vi "2500A and Neocera.vi"() -> ()   [LabVIEW 2010]
uses:
  <vilib>/Utility/file.llb/Write To Spreadsheet File (DBL).vi
  <vilib>/ptbypt/NI_PtbyPt.lvlib
panel:
  in  "AH2500A  GPIB":refnum<visa-resource-name>
  in  "Neocera GPIB":refnum<visa-resource-name>
  in  "Number of\n data points\nto average":i32
  out "Temperature":dbl format="%.3f"
  in  "Save?":bool
  in  "file path (dialog if empty)":path
  out "XY Graph":cluster{dbl[], dbl[]}(graph)
  out "Capacitance":ext format="%#.6g"
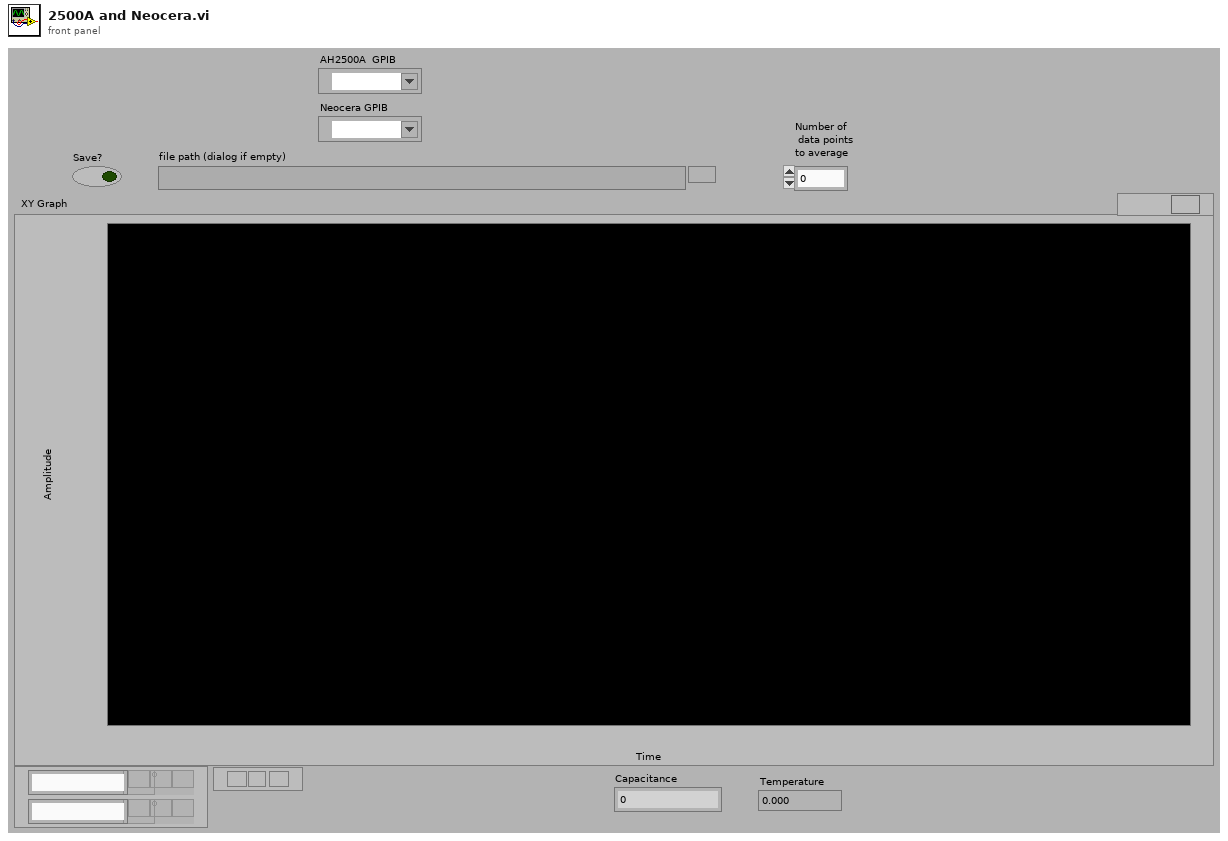
[diagram p1: front panel]
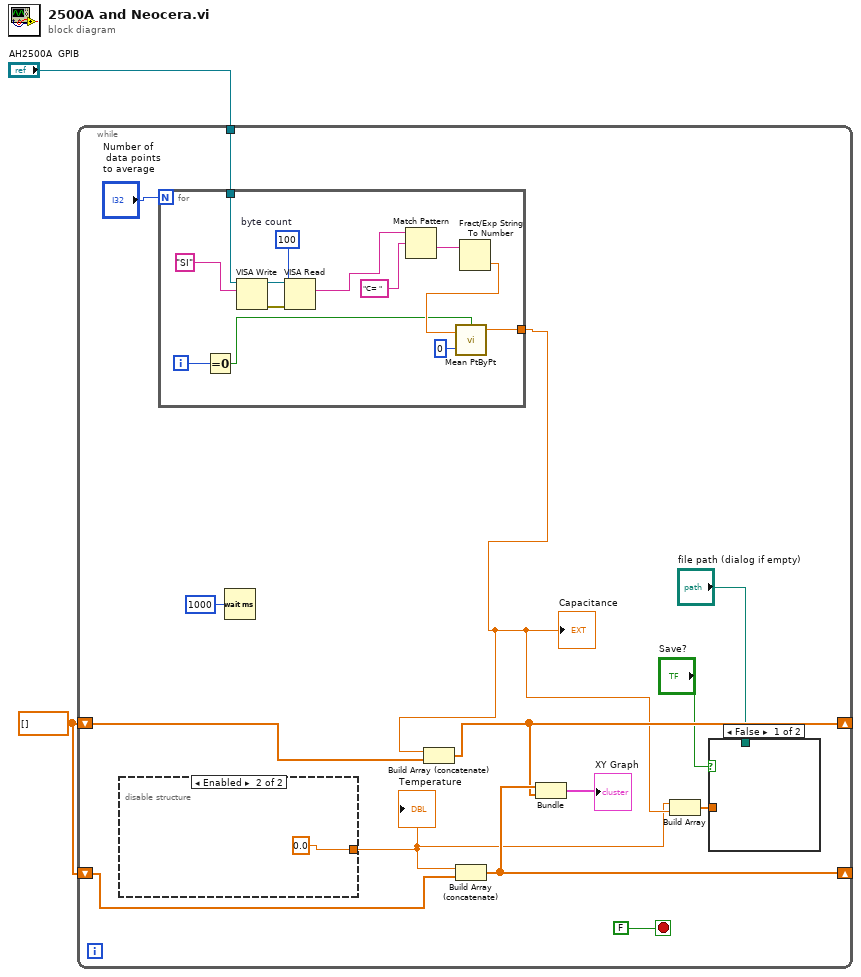
[diagram p0: block diagram]
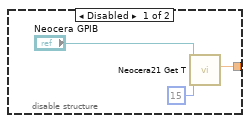
[diagram p2: hidden frame]
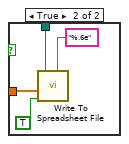
[diagram p3: hidden frame]
diagram:
  w2 = dbl[] []
  n1 = while {
    shift-right: [w11] -> _
    shift-left: w2 -> [w14]
    shift-right: [w10] -> _
    shift-left: w2 -> [w13]
    tunnel: "AH2500A  GPIB" -> [w3]
    stop <- FALSE stop-if-true
    n2 = disable-structure shown="Enabled" {
      disable-tunnel: [w17 0.0] -> w4
      frame Disabled {
        n3 = call "Neocera21 Get T.vi"("Sensor"=i16 15 ("GPIB Adress"), "VISA Resource Name"="Neocera GPIB") -> ("Temperature"=w17:dbl)  [unwired: 6 in, 3 out]
      }
      frame Enabled {
      }
    }
    "Temperature" <- w4
    n4 = for {
      N: "Number of\n data points\nto average" -> [_]
      tunnel: [w30] -> w5
      tunnel: w3 -> [w22]
      i -> [w29]
      w21 = u32 100  # byte count
      n5 = Equal To 0?(x=w29) -> (x = 0?=w28:bool)
      n6 = VISA Write(VISA resource name=w22, write buffer="SI" ("data string")) -> (VISA resource name out=w26:refnum<visa-resource-name>, error out=w25:errorcluster)  [unwired: 1 in, 1 out]
      n7 = VISA Read(VISA resource name=w26, byte count=w21, error in (no error)=w25) -> (read buffer=w23:string)  [unwired: 3 out]
      n8 = Match Pattern(string=w23, regular expression="C= ") -> (after substring=w32:string)  [unwired: 1 in, 3 out]
      n9 = Fract/Exp String To Number(string=w32) -> (number=w31:dbl)  [unwired: 3 in, 1 out]
      n10 = call <vilib>:"Mean PtByPt.vi"("x"=w31, "sample length"=0, "initialize"=w28) -> ("mean"=w30:dbl)  [unwired: 1 in, 1 out]
    }
    "Capacitance" <- w5
    n11 = Wait (ms)(milliseconds to wait=u32 1000) -> ()  [unwired: 1 out]
    n12 = Build Array (concatenate)(w5, w13) -> (w10:dbl[])
    n13 = Build Array (concatenate)(w4, w14) -> (w11:dbl[])
    n14 = Bundle(w11, w10) -> (→"XY Graph":cluster{dbl[], dbl[]})  [unwired: 1 in]
    n15 = Build Array(w4, w5) -> (w9:dbl[])
    n16 = case shown="False" "Save?" {
      tunnel: w9 -> [_ w34]
      tunnel: "file path (dialog if empty)" -> [_ w36]
      frame False {
      }
      frame True {
        n17 = call-poly <vilib>:"Write To Spreadsheet File.vi"("format (%.3f)"="%.6e", "append to file? (new file:F)"=TRUE, "1D data"=w34, "file path (dialog if empty)"=w36) -> ()  [unwired: 4 in, 1 out]
      }
    }
  }
